vi "Status RS485.vi"(8 "error in (no error)":errorcluster, 10 "Internal?":bool, 11 "Huber Unistat 410 Settings":T1 {"Address" min=0 max=99 format="%02.0f"}) -> (0 "error out":errorcluster, 1 "Connection Error":bool, 2 "Running":bool, 3 "Huber Unistat 410 Settings":T1 {"Address" min=0 max=99 format="%02.0f"}, 6 "Temperature":dbl)   [LabVIEW 2018, in "Huber Unistat 410 TCU.lvlib"]
uses:
  Huber Unistat 410 TCU.lvlib
  Huber Unistat 410 RS485 Settings.ctl
  <vilib>/regexp/Match Regular Expression.xnode
panel:
  out "External Temp":string
  out "Internal Temp":string
  out "Setpoint":string
  out "Alarm Status":string
  out "substring":string
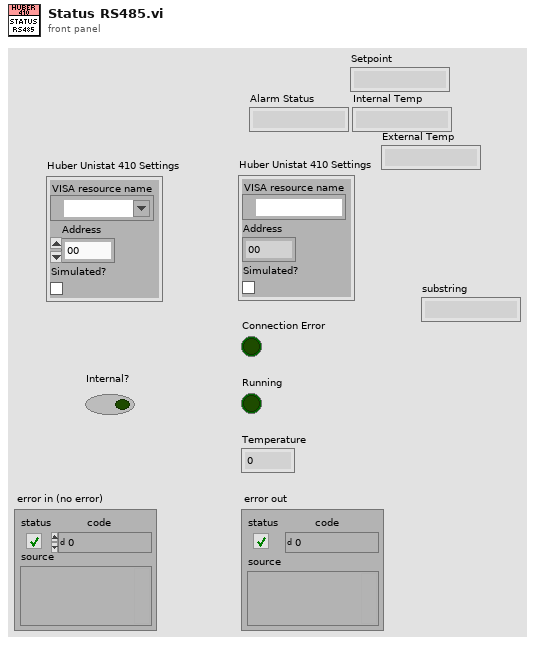
[diagram p1: front panel]
types:
  T1 = typedef "Huber Unistat 410 TCU.lvlib/Huber Unistat 410 RS485 Settings.ctl" = cluster{"VISA resource name":refnum<visa-resource-name>, "Address":i8, "Simulated?":bool}
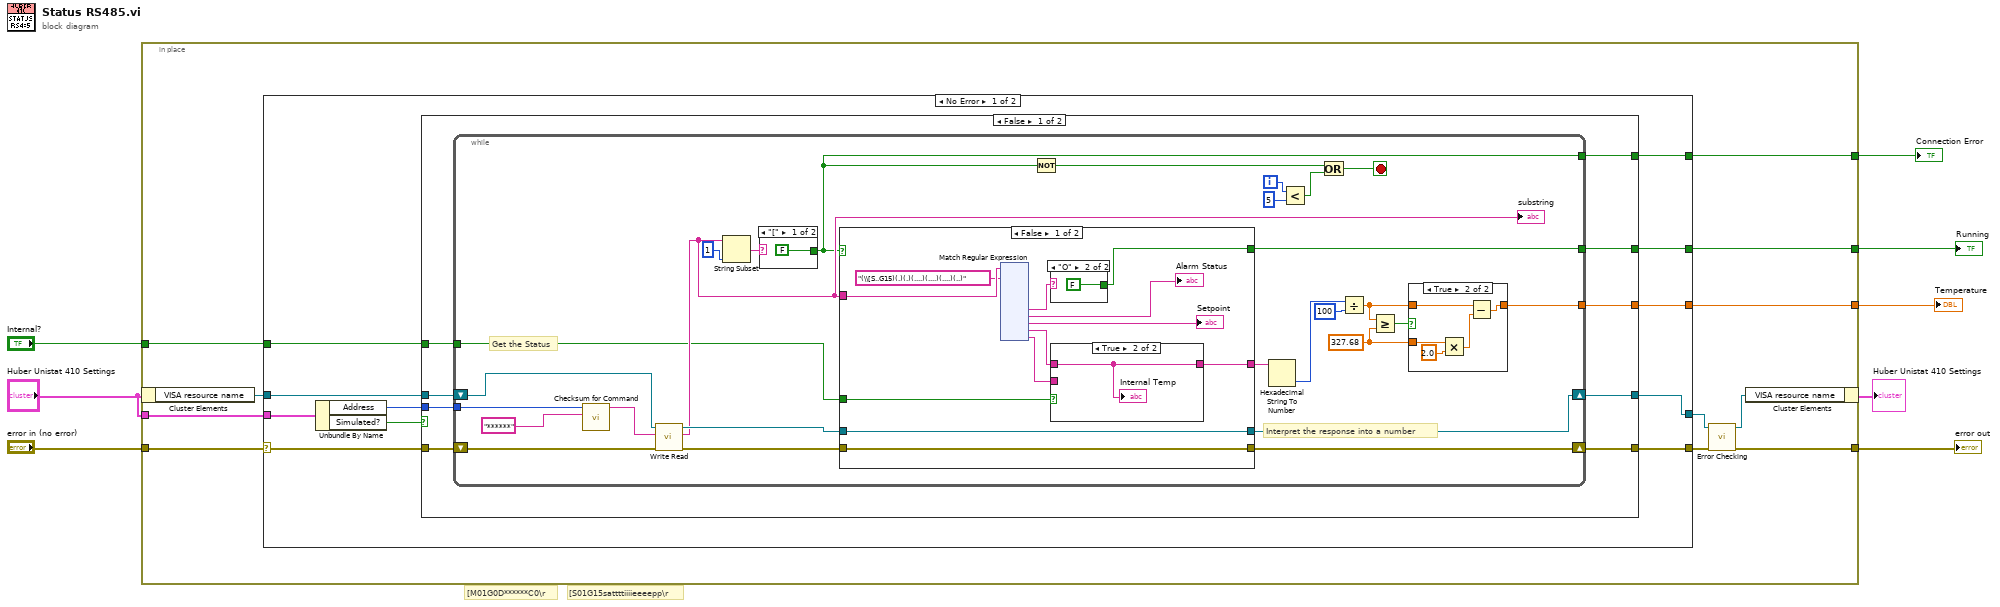
[diagram p0: block diagram]
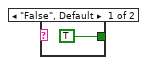
[diagram p3: hidden frame]
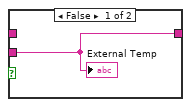
[diagram p4: hidden frame]
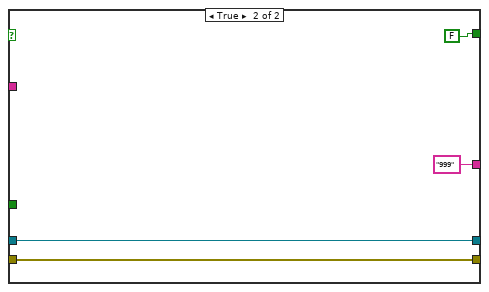
[diagram p5: hidden frame]
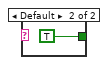
[diagram p6: hidden frame]
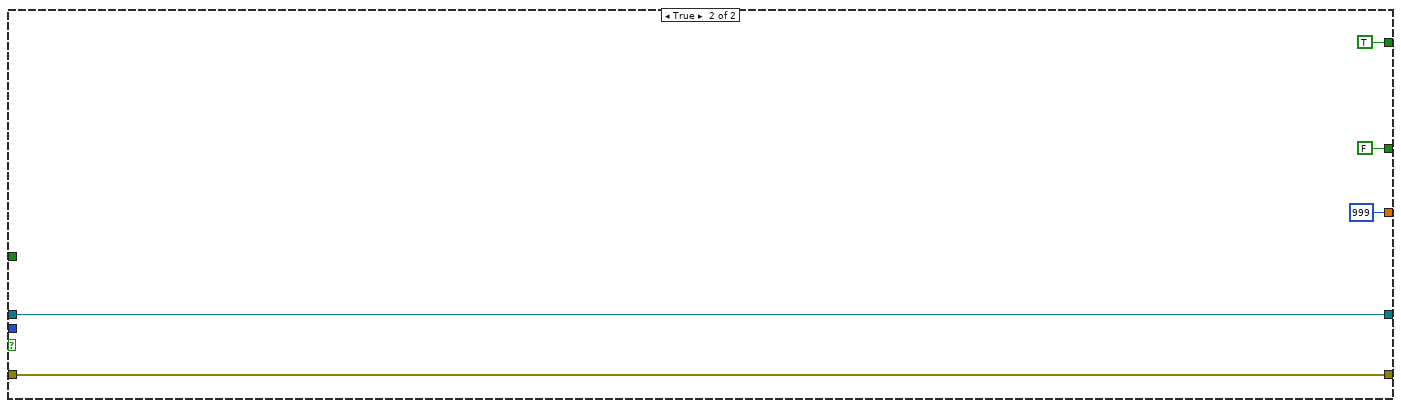
[diagram p7: hidden frame]
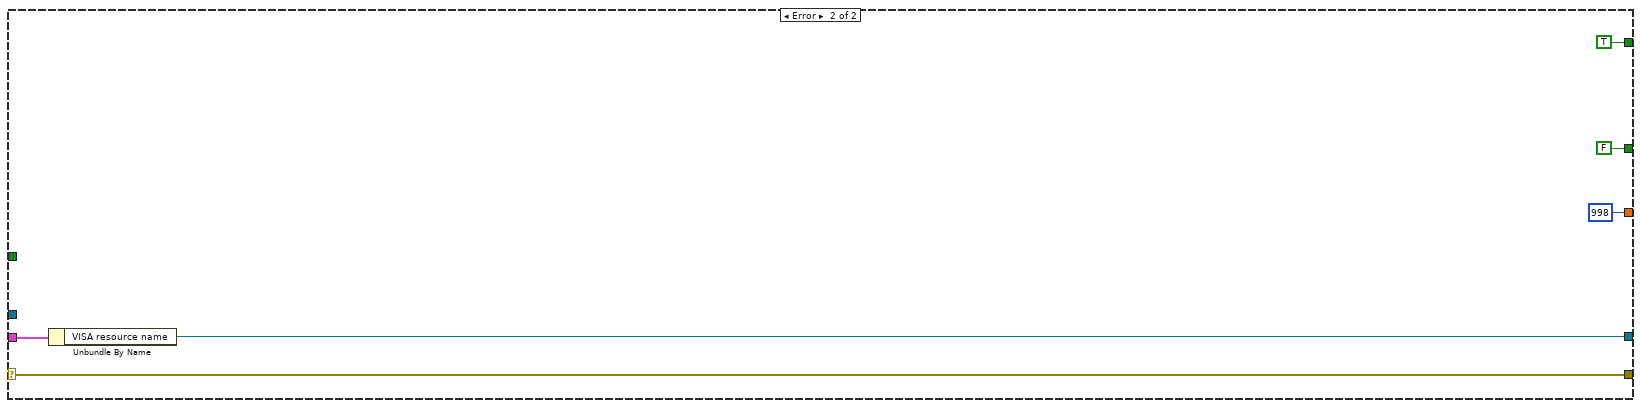
[diagram p8: hidden frame]
diagram:
  # "[S01G15sattttiiiieeeepp\\r"
  # "[M01G0D******C0\\r"
  n1 = in-place {
    in-place-border: "error in (no error)" -> [w19]
    in-place-border: [w16] -> w7
    in-place-border: "Huber Unistat 410 Settings" -> [w15]
    in-place-border: [w14] -> w6
    in-place-border: [w13] -> w5
    in-place-border: [w12] -> w4
    in-place-border: "Internal?" -> [w11]
    n2 = in-place-cluster #1("Huber Unistat 410 Settings") -> ("VISA resource name"=w10:refnum<visa-resource-name>)
    n3 = case shown="No Error" w19 {
      selector: w19 -> [w30 w226]
      tunnel: w15 -> [w28 w225]
      tunnel: [w29 w226] -> w17
      tunnel: [w27 w224] -> w18
      tunnel: [w25 TRUE] -> w14
      tunnel: [w24 FALSE] -> w13
      tunnel: [w23 998] -> w12
      tunnel: w11 -> [w22 _]
      tunnel: w10 -> [w21 _]
      frame No Error {
        n4 = Unbundle By Name(w28) -> ("Address"=w20:i8, "Simulated?"=w26:bool)
        n5 = case shown="False" w26 {
          tunnel: w30 -> [w38 w220]
          tunnel: [w36 w220] -> w29
          tunnel: [w34 w219] -> w27
          tunnel: w21 -> [w39 w219]
          tunnel: [w37 TRUE] -> w25
          tunnel: [w35 FALSE] -> w24
          tunnel: [w32 999] -> w23
          tunnel: w22 -> [w33 _]
          tunnel: w20 -> [w31 _]
          frame False {
            n6 = while {
              tunnel: [w52] -> w37
              tunnel: [w59] -> w35
              tunnel: w33 -> [w50]
              tunnel: [w44] -> w32
              shift-right: [w58] -> w34
              shift-left: w39 -> [w65]
              shift-right: [w61] -> w36
              shift-left: w38 -> [w64]
              tunnel: w31 -> [w42]
              i -> [w53]
              stop <- w51 stop-if-true
              w45 = 327.68 ("y")
              # "Interpret the response into a number"
              # "Get the Status"
              n7 = call "Checksum for Command.vi"("Message"="******" ("string"), "Address"=w42) -> ("Formated Message"=w40:string)  [unwired: 9 in]
              n8 = call "Write Read.vi"("error in (no error)"=w64, "write string"=w40, "VISA Refnum in"=w65) -> ("error out"=w62:errorcluster, "read string"=w57:string, "VISA Refnum out"=w60:refnum<visa-resource-name>)  [unwired: 6 in]
              "substring" <- w57
              n9 = String Subset(string=w57, length (rest)=1 ("length (rest)")) -> (substring=w63:string)  [unwired: 1 in]
              n10 = case shown="\"[\"" w63 {
                tunnel: [FALSE TRUE] -> w52
                frame "[" {
                }
                frame Default {
                }
              }
              n11 = case shown="False" w52 {
                tunnel: w57 -> [w84 _]
                tunnel: [w77 "999" ("whole match")] -> w43
                tunnel: w62 -> [w76 w212]
                tunnel: [w76 w212] -> w61
                tunnel: w60 -> [w75 w210]
                tunnel: [w73 FALSE] -> w59
                tunnel: [w75 w210] -> w58
                tunnel: w50 -> [w80 _]
                frame False {
                  n12 = xnode "Match Regular Expression"("input string"=w84, "regular expression"="(\\[S..G15)(.)(.)(....)(....)(....)(..)") -> ("submatch 2"=w74:string, "submatch 3"=→"Alarm Status":string, "submatch 4"=→"Setpoint":string, "submatch 5"=w79:string, "submatch 6"=w78:string)  [unwired: 4 in, 6 out]
                  n13 = case shown="\"O\"" w74 {
                    tunnel: [TRUE FALSE] -> w73
                    frame "False", Default {
                    }
                    frame "O" {
                    }
                  }
                  n14 = case shown="True" w80 {
                    tunnel: w79 -> [_ w88]
                    tunnel: w78 -> [w87 _]
                    tunnel: [w87 w88] -> w77
                    frame False {
                      "External Temp" <- w87
                    }
                    frame True {
                      "Internal Temp" <- w88
                    }
                  }
                }
                frame True {
                }
              }
              n15 = Not(x=w52) -> (.not. x?=w55:bool)
              n16 = Hexadecimal String To Number(string=w43) -> (number=w46:u32)  [unwired: 2 in, 1 out]
              n17 = Less?(x=w53, y=5) -> (x < y?=w54:bool)
              n18 = Or(x=w55, y=w54) -> (x .or. y?=w51:bool)
              n19 = Divide(x=w46, y=100) -> (x/y=w47:dbl)
              n20 = Greater Or Equal?(x=w47, y=w45) -> (x >= y?=w48:bool)
              n21 = case shown="True" w48 {
                tunnel: w47 -> [w67 w72]
                tunnel: [w67 w68] -> w44
                tunnel: w45 -> [_ w71]
                frame False {
                }
                frame True {
                  n22 = Multiply(x=w71, y=2.0) -> (x*y=w69:dbl)
                  n23 = Subtract(x=w72, y=w69) -> (x-y=w68:dbl)
                }
              }
            }
          }
          frame True {
          }
        }
      }
      frame Error {
        n24 = Unbundle By Name(w225) -> ("VISA resource name"=w224:refnum<visa-resource-name>)
      }
    }
    n25 = call "Error Checking.vi"("error in (no error)"=w17, "VISA resource name"=w18) -> ("error out"=w16:errorcluster, "VISA resource name"=w9:refnum<visa-resource-name>)  [unwired: 7 in, 1 out]
    n26 = in-place-cluster #1("VISA resource name"=w9) -> (→"Huber Unistat 410 Settings":T1)
  }
  "error out" <- w7
  "Connection Error" <- w6
  "Running" <- w5
  "Temperature" <- w4
